vi "splash_screen_update_msg_v1.0.vi"(8 "error in (no error)":errorcluster, 11 "message in":string="Loading DAQ resources...") -> (0 "error out":errorcluster)   [LabVIEW 2025]
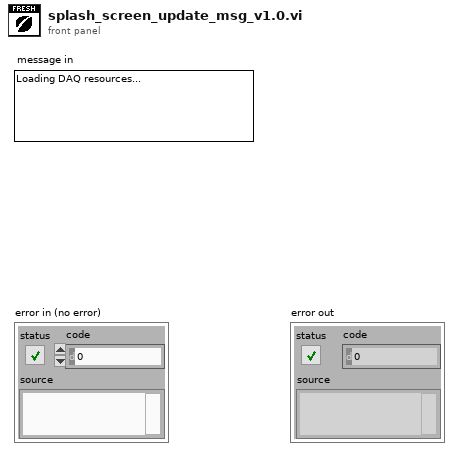
[diagram p1: front panel]
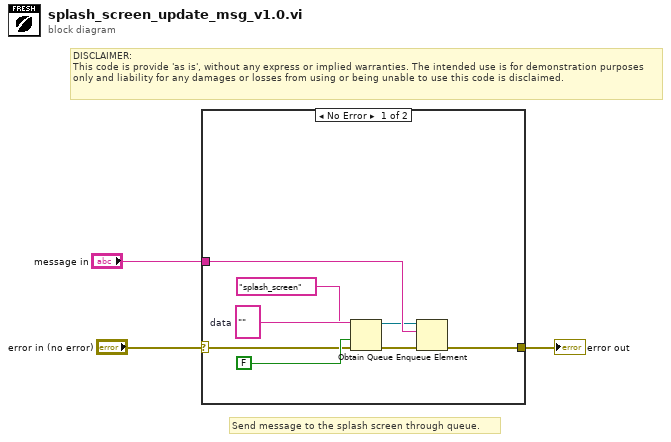
[diagram p0: block diagram]
diagram:
  # "Send message to the splash screen through queue."
  # "DISCLAIMER:\nThis code is provide 'as is', without any express or implied warranties. The intended use is for demonstration purposes only and liability for any damages or losses from using or being unable to use this code is disclaimed."
  n1 = case shown="No Error" "error in (no error)" {
    selector: "error in (no error)" -> [w4 w12]
    tunnel: [w5 w12] -> w2
    tunnel: "message in" -> [w11 _]
    frame No Error {
      w10 = ""  # data
      n2 = Obtain Queue(name (unnamed)="splash_screen", element data type=w10, create if not found? (T)=FALSE, error in (no error)=w4) -> (queue out=w7:refnum<queue>, error out=w8:errorcluster)  [unwired: 1 in, 1 out]
      n3 = Enqueue Element(queue=w7, element=w11, error in (no error)=w8) -> (error out=w5:errorcluster)  [unwired: 1 in, 2 out]
    }
    frame Error {
    }
  }
  "error out" <- w2
